vi "set_settings_cluster.vi"(8 "error in (no error)":errorcluster, 10 "settings cluster in":variant, 11 "GenericPlugin in":refnum<class "ImagingModeMG090624Camera.lvclass">) -> (0 "error out":errorcluster, 3 "GenericPlugin out":refnum<class "ImagingModeMG090624Camera.lvclass">)   [LabVIEW 2010, in "ImagingModeMG090624Camera.lvclass"]
uses:
  ImagingModeMG090624Camera.lvclass
  ImagingModeMG090624Camera.lvclass/ImagingModeMG090624Camera.ctl
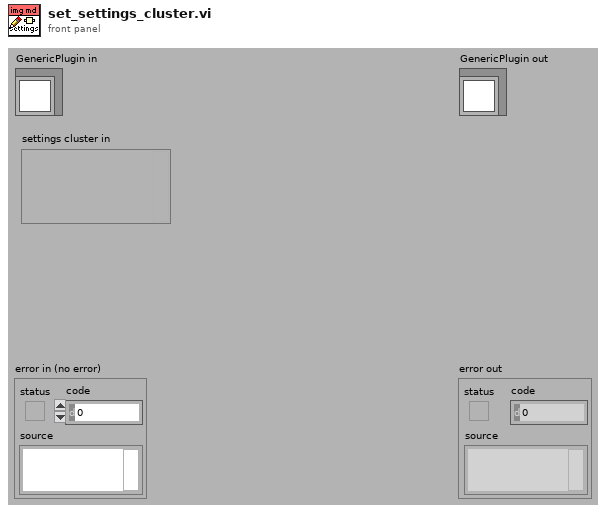
[diagram p1: front panel]
types:
  T1 = typedef "ImagingModeMG090624Camera.lvclass/settings_cluster.ctl" = cluster{"x resolution ":i32, "y resolution":i32, "frame rate":dbl[unit], "number of frames":i32}
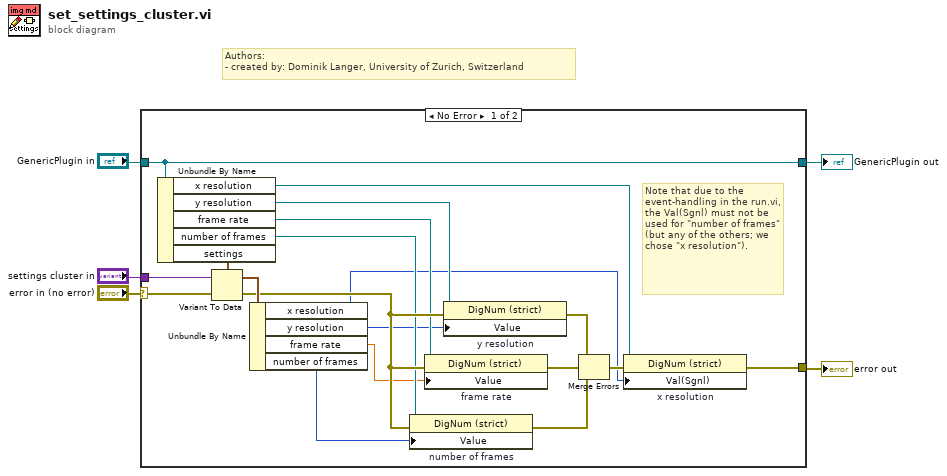
[diagram p0: block diagram]
diagram:
  # "Authors: \n- created by: Dominik Langer, University of Zurich, Switzerland"
  n1 = case shown="No Error" "error in (no error)" {
    selector: "error in (no error)" -> [w8 w26]
    tunnel: [w23 w26] -> w4
    tunnel: [w6 w25] -> w2
    tunnel: "GenericPlugin in" -> [w6 w25]
    tunnel: "settings cluster in" -> [w7 _]
    frame No Error {
      # "Note that due to the event-handling in the run.vi, the Val(Sgnl) must not be used for \"number of frames\" (but any of the others; we chose \"x resolution\")."
      n2 = Unbundle By Name(w6) -> ("x resolution"=w15:refnum<vi>, "y resolution"=w13:refnum<vi>, "frame rate"=w14:refnum<vi>, "number of frames"=w17:refnum<vi>, "settings"=w9:T1)
      n3 = Variant To Data(error in=w8, Variant=w7, type=w9) -> (error out=w21:errorcluster, data=w24:T1)
      n4 = Unbundle By Name(w24) -> ("x resolution"=w10:i32, "y resolution"=w11:i32, "frame rate"=w12:dbl[unit], "number of frames"=w16:i32)
      n5 = property on="number of frames" class="DigNum (strict)"(reference=w17, error in=w21, "Value"=w16) -> (error out=w18:errorcluster)  [unwired: 1 out]
      n6 = property on="frame rate" class="DigNum (strict)"(reference=w14, error in=w21, "Value"=w12) -> (error out=w19:errorcluster)  [unwired: 1 out]
      n7 = property on="y resolution" class="DigNum (strict)"(reference=w13, error in=w21, "Value"=w11) -> (error out=w20:errorcluster)  [unwired: 1 out]
      n8 = Merge Errors(w20, w19, w18) -> (w22:errorcluster)
      n9 = property on="x resolution" class="DigNum (strict)"(reference=w15, error in=w22, "Val(Sgnl)"=w10) -> (error out=w23:errorcluster)  [unwired: 1 out]
    }
    frame Error {
    }
  }
  "error out" <- w4
  "GenericPlugin out" <- w2
